vi "Add Entity.vi"(8 "error in (no error)":errorcluster, 10 "Conditum:Entity":refnum<class "Entity.lvclass">, 11 "Entity Collection in":refnum<class "Entity Collection.lvclass">) -> (0 "error out":errorcluster, 3 "Entity Collection out":refnum<class "Entity Collection.lvclass">)   [LabVIEW 2020, in "Conditum.lvlib" / "Columns.lvlib" / "Entity Collection.lvclass"]
uses:
  Entity Collection.lvclass
  Entity/Entity.lvclass
  Entity Collection.lvclass/Entity Collection.ctl
  Entity Sort.ctl
  Entity/Entity.lvclass/Entity.ctl
  ID/ID.lvclass/ID.ctl
  <vilib>/Utility/miscctls.llb/LVMapReplaceAction.ctl
  ID/Get.vi
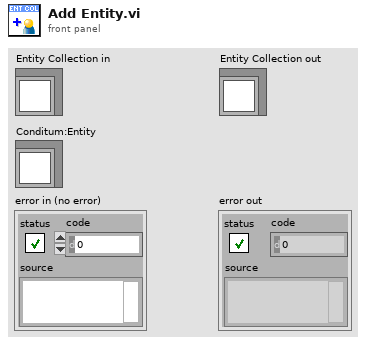
[diagram p1: front panel]
types:
  T1 = typedef "Conditum.lvlib/Columns.lvlib/Entity Collection.lvclass/Entity Sort.ctl" = cluster{"Order":u64, "Entity":refnum<class "Entity.lvclass">}
  T2 = typedef "LVMapReplaceAction.ctl" = enum32{"Modify Entry only if found", "Add or Modify Entry", "Delete Entry"}
  T3 = typedef "Conditum.lvlib/Entity ID.ctl" = i64
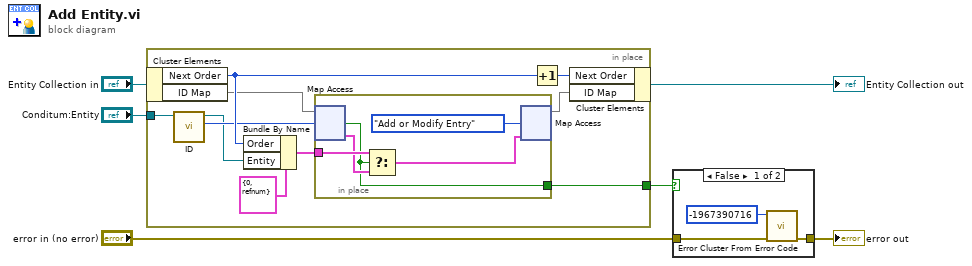
[diagram p0: block diagram]
diagram:
  n1 = in-place {
    in-place-border: "Conditum:Entity" -> [w16]
    in-place-border: [w8] -> w1
    n2 = in-place-cluster #1("Entity Collection in") -> ("Next Order"=w13:u64, "ID Map"=w12:map{T3, T1})
    n3 = call "ID.vi"("Entity in"=w16) -> ("ID"=w11:T3, "Entity out"=w10:refnum<class "Entity.lvclass">)  [unwired: 9 in]
    n4 = Bundle By Name(cluster=T1 {"Order"=0, "Entity"=refnum} ("Entity Sort"), "Order"=w13, "Entity"=w10) -> (w9:T1)
    n5 = in-place {
      in-place-border: w9 -> [w21]
      in-place-border: [w17] -> w8
      n6 = in-place-map #2(w12, w11) -> (w20:T1, w17:bool)  [unwired: 1 in]
      n7 = Select(t=w21, s=w17, f=w20) -> (s? t:f=w19:T1)
      n8 = in-place-map #2(w19, LVMapReplaceAction."Add or Modify Entry" ("action")) -> (w7:map{T3, T1})  [unwired: 2 out]
    }
    n9 = Increment(x=w13) -> (x+1=w15:u64)
    n10 = in-place-cluster #1("Next Order"=w15, "ID Map"=w7) -> (→"Entity Collection out":refnum<class "Entity Collection.lvclass">)
  }
  n11 = case shown="False" w1 {
    tunnel: "error in (no error)" -> [w24 w25]
    tunnel: [w23 w25] -> w2
    frame False {
      n12 = call <vilib>:"Error Cluster From Error Code.vi"("error in (no error)"=w24, "error code (0)"=-1967390716) -> ("error out"=w23:errorcluster)  [unwired: 7 in]
    }
    frame True {
    }
  }
  "error out" <- w2
